vi "4Pi 4Pi Modes - Make Mirror Pattern.vi"(0 "Coefficients":T1, 2 "Flat On?":bool, 5 "Astig Coeffs":T1, 9 "Flats":dbl[](array[numeric]), 11 "Control Matrix":dbl[][](array[numeric])) -> (8 "Pixel Value U (-1 to 1)":dbl[](array[numeric]), 15 "error":i32)   [LabVIEW 2016]
uses:
  4Pi 4Pi Modes - Controls/4Pi 4Pi Modes - Mirror Modes.ctl
  <vilib>/Analysis/baseanly.llb/A x Vector.vi
  <vilib>/Analysis/NI_AALBase.lvlib
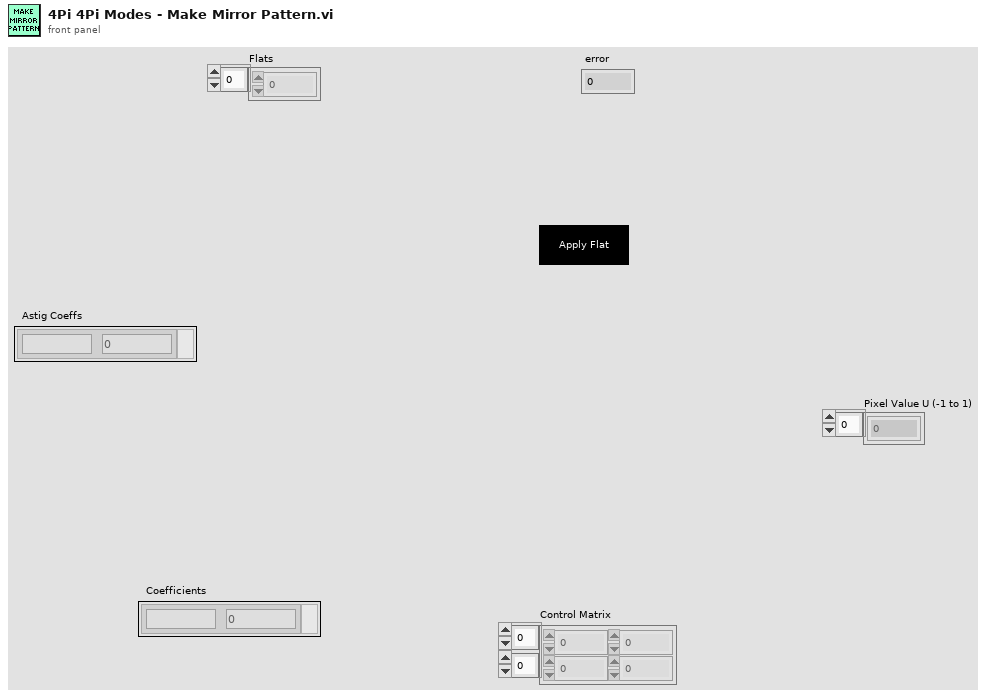
[diagram p1: front panel]
types:
  T1 = typedef "4Pi 4Pi Modes - Mirror Modes.ctl" = cluster{"Mode":string, "Amplitude":dbl}[]
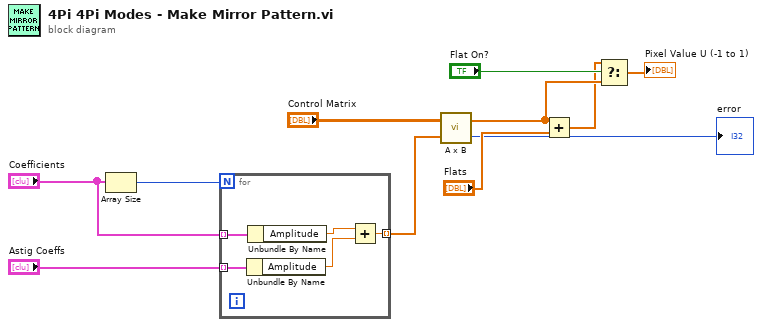
[diagram p0: block diagram]
diagram:
  n1 = Array Size(array="Coefficients") -> (size(s)=w10:i32)
  n2 = for {
    N: w10 -> [_]
    tunnel: "Coefficients" -> [w16] mode=indexing
    tunnel: [w14] -> w7 mode=indexing
    tunnel: "Astig Coeffs" -> [w15] mode=indexing
    n3 = Unbundle By Name(w15) -> ("Amplitude"=w12:dbl)
    n4 = Unbundle By Name(w16) -> ("Amplitude"=w13:dbl)
    n5 = Add(x=w13, y=w12) -> (x+y=w14:dbl)
  }
  n6 = call-poly <vilib>:"A x B.vi"("Vector"=w7, "A"="Control Matrix") -> ("error"=→"error":i32, "A x Vector"=w5:dbl[])
  n7 = Add(x=w5, y="Flats") -> (x+y=w4:dbl[])
  n8 = Select(t=w4, s="Flat On?", f=w5) -> (s? t:f=→"Pixel Value U (-1 to 1)":dbl[])
